vi "Scan Audio Devices.vi"(6 "error in (no error)":errorcluster) -> (0 "error out":errorcluster, 4 "Number of Speakers":i32, 5 "Number of Mics":i32)   [LabVIEW 2020]
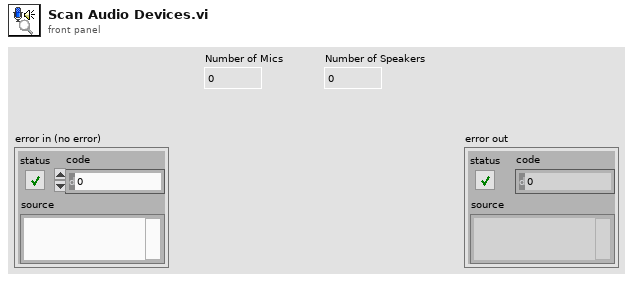
[diagram p1: front panel]
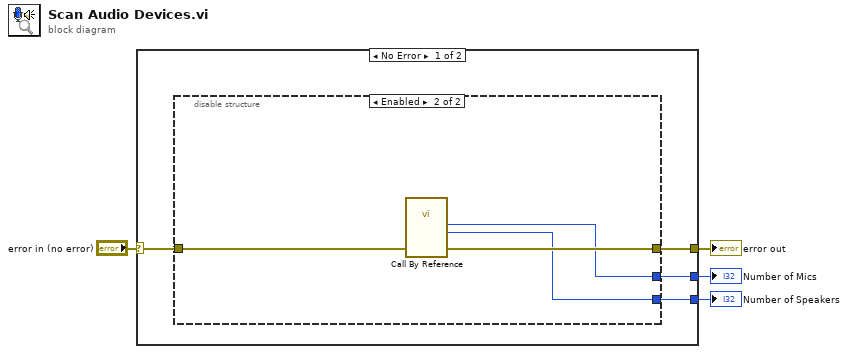
[diagram p0: block diagram]
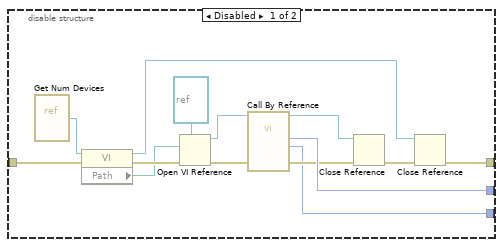
[diagram p2: hidden frame]
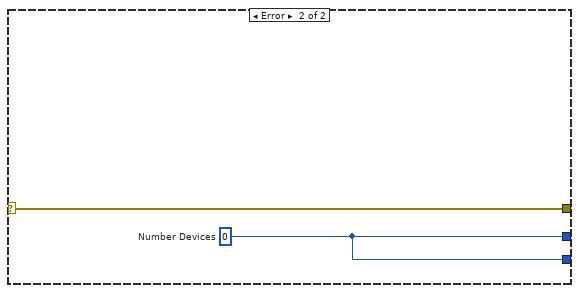
[diagram p3: hidden frame]
diagram:
  n1 = case shown="No Error" "error in (no error)" {
    selector: "error in (no error)" -> [w7 w28]
    tunnel: [w8 w27] -> w4
    tunnel: [w5 w28] -> w2
    tunnel: [w6 w27] -> w1
    frame No Error {
      n2 = disable-structure shown="Enabled" {
        disable-tunnel: [w22 w24] -> w8
        disable-tunnel: w7 -> [w21 w26]
        disable-tunnel: [w13 w23] -> w6
        disable-tunnel: [w10 w25] -> w5
        frame Disabled {
          n3 = vi-ref <vilib>:"Get Num Devices.vi"() -> (w17:refnum<vi>)
          n4 = property class="VI"(reference=w17, error in=w21) -> (reference out=w9:refnum<vi>, error out=w20:errorcluster, "Path"=w18:path)
          n5 = Open VI Reference(type specifier VI Refnum (for type only)=refnum<vi> refnum, vi path=w18, error in (no error)=w20) -> (vi reference=w16:refnum<vi>, error out=w19:errorcluster)  [unwired: 3 in]
          n6 = call-by-ref "?"(reference=w16, "error in (no error)"=w19) -> (reference out=w11:refnum<vi>, "error out"=w14:errorcluster, "Number of Output Devices"=w13:i32, "Number of Input Devices"=w22:i32)  [unwired: 9 in, 1 out]
          n7 = Close Reference(reference=w11, error in (no error)=w14) -> (error out=w12:errorcluster)
          n8 = Close Reference(reference=w9, error in (no error)=w12) -> (error out=w10:errorcluster)
        }
        frame Enabled {
          n9 = call-by-ref "?"("error in (no error)"=w26) -> ("error out"=w25:errorcluster, "Number of Output Devices"=w23:i32, "Number of Input Devices"=w24:i32)  [unwired: 10 in, 2 out]
        }
      }
    }
    frame Error {
      w27 = 0  # Number Devices
    }
  }
  "Number of Mics" <- w4
  "error out" <- w2
  "Number of Speakers" <- w1
